vi "NCS_AmpPh_v2.vi"(6 "Rx Channel Tone":dbl=0.45000000000000007 format="%0.2f", 8 "IQ":cdb[](array[numeric]), 9 "data":cdb[][](array[numeric]), 10 "Sampling Rate":i32=500, 11 "Coerced Rx IQ Rate":dbl) -> (0 "Phase DownSampled":dbl[](array[numeric]), 1 "Amp DownSampled":dbl[](array[numeric]), 2 "Phase":dbl[](array[numeric]), 3 "Amplitude":dbl[](array[numeric]))   [LabVIEW 2016]
uses:
  <vilib>/Analysis/3filter.llb/Filter Passband Type.ctl
  <vilib>/Analysis/3filter.llb/Butterworth Filter (CDB).vi
  <vilib>/Analysis/3filter.llb/Butterworth Filter (DBL).vi
  <vilib>/Analysis/NI_AALBase.lvlib
  <vilib>/Analysis/NI_AALPro.lvlib
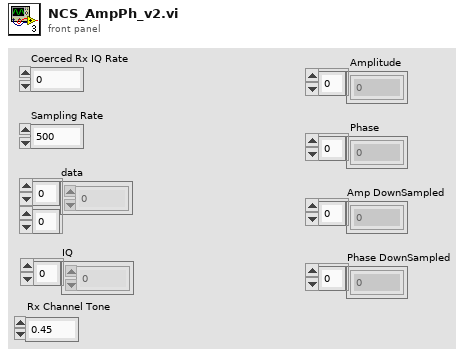
[diagram p1: front panel]
types:
  T1 = typedef "NI_AALBase.lvlib/Filter Passband Type.ctl" = enum32{"Lowpass", "Highpass", "Bandpass", "Bandstop"}
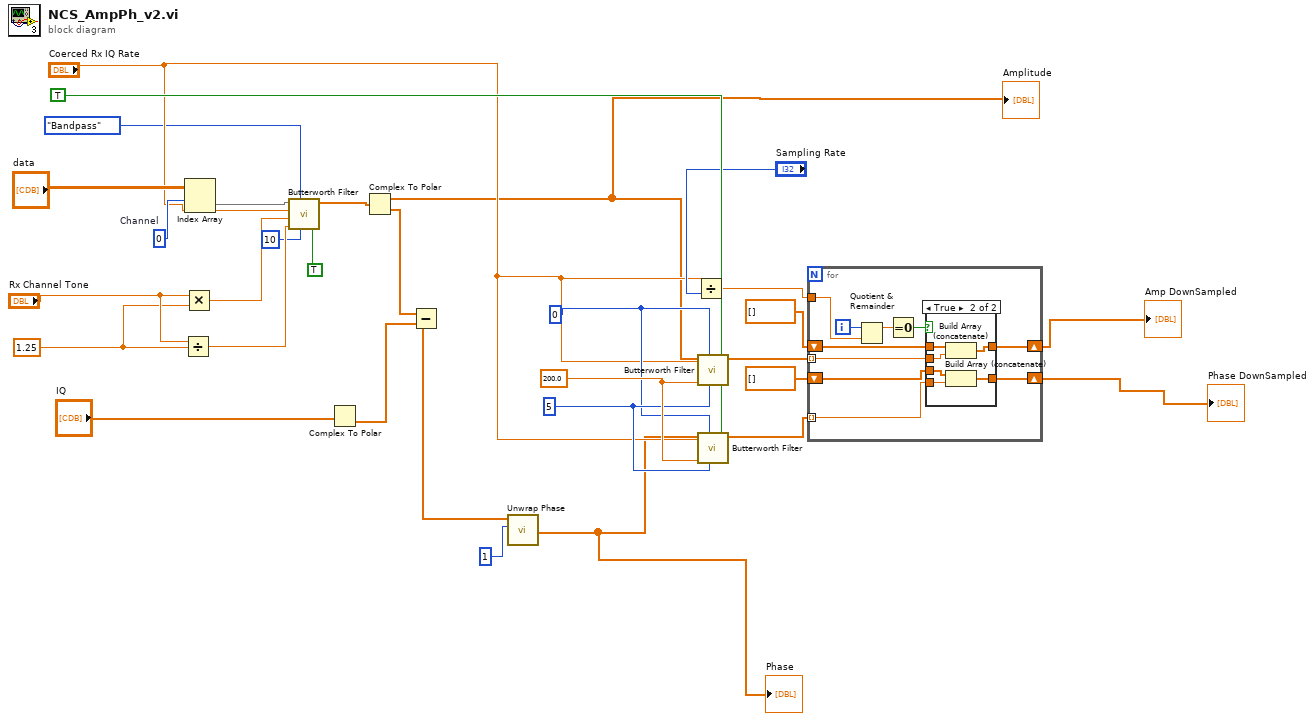
[diagram p0: block diagram]
diagram:
  w12 = 1.25
  w18 = 0  # Channel
  w27 = 5 ("order1")
  w30 = 200.0 ("Low-Pass Freq")
  w28 = TRUE
  w26 = 0
  n1 = Divide(x="Rx Channel Tone", y=w12) -> (x/y=w11:dbl)
  n2 = Multiply(x="Rx Channel Tone", y=w12) -> (x*y=w14:dbl)
  n3 = Index Array(array="data", index (row)=w18) -> (element=w7:cdb[])  [unwired: 1 in]
  n4 = call-poly <vilib>:"Butterworth Filter.vi"("init/cont (init:F)"=TRUE, "order"=10, "filter type"=Filter_Passband_Type."Bandpass", "low cutoff freq: fl"=w11, "high cutoff freq: fh"=w14, "sampling freq: fs"="Coerced Rx IQ Rate", "X"=w7) -> ("Filtered X"=w6:cdb[])  [unwired: 1 in, 1 out]
  n5 = Complex To Polar(r * e^(i*theta)="IQ") -> (theta=w23:dbl[])  [unwired: 1 out]
  n6 = Complex To Polar(r * e^(i*theta)=w6) -> (r=w3:dbl[], theta=w25:dbl[])
  "Amplitude" <- w3
  n7 = Subtract(x=w25, y=w23) -> (x-y=w16:dbl[])
  n8 = call <vilib>:"Unwrap Phase.vi"("phase unit"=1 ("y"), "Phase"=w16) -> ("Unwrapped Phase"=w2:dbl[])  [unwired: 8 in, 1 out]
  "Phase" <- w2
  n9 = Divide(x="Coerced Rx IQ Rate", y="Sampling Rate") -> (x/y=w21:dbl)
  n10 = call-poly <vilib>:"Butterworth Filter.vi"("init/cont (init:F)"=w28, "order"=w27, "filter type"=w26, "low cutoff freq: fl"=w30, "sampling freq: fs"="Coerced Rx IQ Rate", "X"=w3) -> ("Filtered X"=w5:dbl[])  [unwired: 2 in, 1 out]
  n11 = call-poly <vilib>:"Butterworth Filter.vi"("init/cont (init:F)"=w28, "order"=w27, "filter type"=w26, "low cutoff freq: fl"=w30, "sampling freq: fs"="Coerced Rx IQ Rate", "X"=w2) -> ("Filtered X"=w1:dbl[])  [unwired: 2 in, 1 out]
  n12 = for {
    tunnel: w5 -> [w41] mode=indexing
    shift-right: [w39] -> w31
    shift-left: dbl[] [] -> [w40]
    tunnel: w21 -> [w35]
    shift-right: [w33] -> w4
    shift-left: dbl[] [] -> [w34]
    tunnel: w1 -> [w32] mode=indexing
    i -> [w38]
    n13 = Quotient & Remainder(x=w38, y=w35) -> (x-y*floor(x/y)=w36:dbl)  [unwired: 1 out]
    n14 = Equal To 0?(x=w36) -> (x = 0?=w37:bool)
    n15 = case shown="True" w37 {
      tunnel: w41 -> [_ w49]
      tunnel: w40 -> [w43 w48]
      tunnel: [w43 w47] -> w39
      tunnel: w34 -> [w42 w46]
      tunnel: [w42 w45] -> w33
      tunnel: w32 -> [_ w44]
      frame False {
      }
      frame True {
        n16 = Build Array (concatenate)(w48, w49) -> (w47:dbl[])
        n17 = Build Array (concatenate)(w46, w44) -> (w45:dbl[])
      }
    }
  }
  "Amp DownSampled" <- w31
  "Phase DownSampled" <- w4
